vi "value2range_ADC.vi"(2 "Current [A]":dbl) -> (1 "Limited current [A]":dbl, 3 "Negative":bool, 4 "Positive or zero":bool, 5 "Range limit (unsigned) [A]":dbl, 6 "Range limit (signed) [A]":dbl, 7 "Range [-]":i32, 8 "Positive":bool, 9 "Overflow":bool)   [LabVIEW 2020, in "Datron D4xxx.lvlib"]
doc: "This VI returns range for entered current value."
uses:
  Datron D4xxx.lvlib
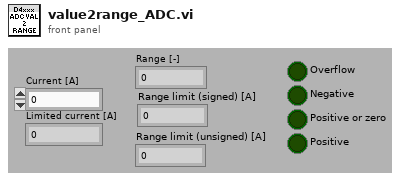
[diagram p1: front panel]
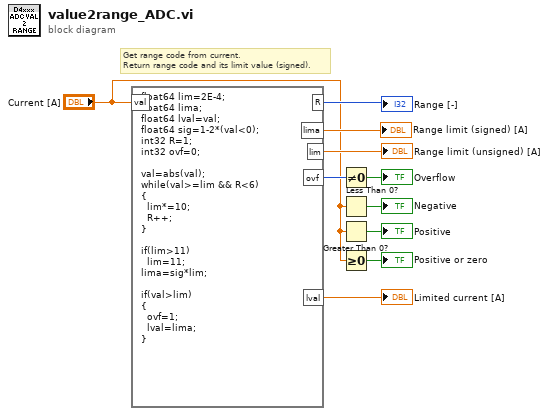
[diagram p0: block diagram]
diagram:
  # "Get range code from current.\nReturn range code and its limit value (signed)."
  n1 = formula code="float64 lim=2E-4;\nfloat64 lima;\nfloat64 lval=val;\nfloat64 sig=1-2*(val<0);\nint32 R=1;\nint32 ovf=0;\n\nval=abs(val);\nwhile(val>=lim && R<6)\n{\n  lim*=10;\n  R++;\n}\n\nif(lim>11)\n  lim=11;\nlima=sig*lim;\n\nif(val>lim)\n{\n  ovf=1;\n  lval=lima;\n}"("val"="Current [A]") -> ("R"=→"Range [-]":i32, "lima"=→"Range limit (signed) [A]":dbl, "lim"=→"Range limit (unsigned) [A]":dbl, "ovf"=w7:i32, "lval"=→"Limited current [A]":dbl)
  n2 = Not Equal To 0?(x=w7) -> (x != 0?=→"Overflow":bool)
  n3 = Less Than 0?(x="Current [A]") -> (x < 0?=→"Negative":bool)
  n4 = Greater Than 0?(x="Current [A]") -> (x > 0?=→"Positive":bool)
  n5 = Greater Or Equal To 0?(x="Current [A]") -> (x >= 0?=→"Positive or zero":bool)
